vi "AssertXPathConnectorPanesMatchTemplateFiles.vi"(8 "error in (no error)":errorcluster, 9 "absolute custom device xml file":path, 10 "connector pane templates":T1[](array[typedef]), 11 "TestCase in":refnum<class "TestCase.lvclass">) -> (0 "error out":errorcluster, 3 "TestCase out":refnum<class "TestCase.lvclass">)   [LabVIEW 2015, in "VeriStandTestCase.lvclass"]
uses:
  VeriStandTestCase.lvclass
  <vilib>/addons/_JKI Toolkits/VI Tester/TestCase.llb/TestCase.lvclass
  ConnectorPaneTemplate.ctl
  <vilib>/xml/Load XML File.vi
  <userlib>/_OpenG.lib/array/array.llb/Remove Duplicates from 1D Array (String)__ogtk.vi
  <vilib>/xml/Close Reference(Node).vi
  <vilib>/xml/NI_XML.lvlib
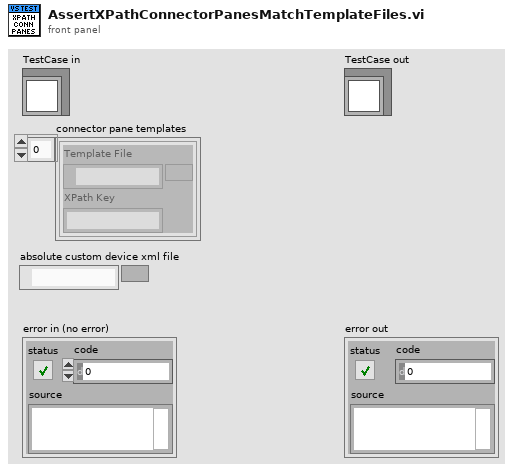
[diagram p1: front panel]
types:
  T1 = typedef "VeriStandTestCase.lvclass/ConnectorPaneTemplate.ctl" = cluster{"Template File":path, "XPath Key":string}
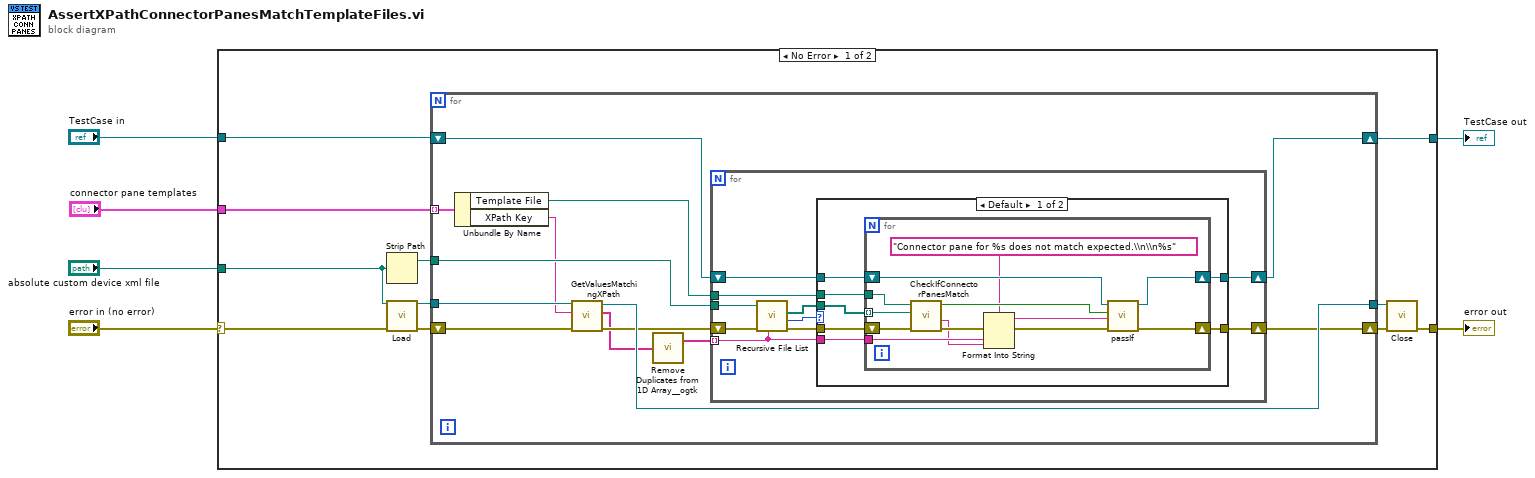
[diagram p0: block diagram]
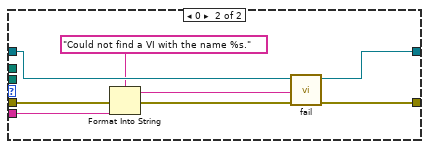
[diagram p2: hidden frame]
diagram:
  n1 = case shown="No Error" "error in (no error)" {
    selector: "error in (no error)" -> [w8 w70]
    tunnel: "absolute custom device xml file" -> [w16 _]
    tunnel: [w15 w69] -> w5
    tunnel: "TestCase in" -> [w13 w69]
    tunnel: [w11 w70] -> w3
    tunnel: "connector pane templates" -> [w7 _]
    frame No Error {
      n2 = Strip Path(path=w16) -> (stripped path=w17:path)  [unwired: 1 out]
      n3 = call-poly <vilib>:"Load.vi"("path to XML document"=w16, "error in (no error)"=w8) -> ("DOM document out"=w10:refnum<k20>, "error out"=w9:errorcluster)  [unwired: 11 in, 1 out]
      n4 = for {
        shift-right: [w23] -> w14
        shift-left: w9 -> [w29]
        tunnel: w10 -> [w30]
        tunnel: [w28] -> w12
        tunnel: w7 -> [w20] mode=indexing
        shift-right: [w27] -> w15
        shift-left: w13 -> [w26]
        tunnel: w17 -> [w25]
        n5 = Unbundle By Name(w20) -> ("Template File"=w18:path, "XPath Key"=w19:string)
        n6 = call "GetValuesMatchingXPath.vi"("error in (no error)"=w29, "XPath"=w19, "XML refnum in"=w30) -> ("error out"=w24:errorcluster, "Values"=w22:string[], "XML refnum out"=w28:refnum<k20>)  [unwired: 6 in]
        n7 = call-poly <userlib>:"Remove Duplicates from 1D Array__ogtk.vi"("Input Array"=w22) -> ("Output Array"=w21:string[])  [unwired: 1 out]
        n8 = for {
          shift-right: [w38] -> w23
          shift-left: w24 -> [w40]
          tunnel: w21 -> [w34] mode=indexing
          tunnel: w25 -> [w39]
          tunnel: w18 -> [w37]
          shift-right: [w35] -> w27
          shift-left: w26 -> [w36]
          n9 = call <vilib>:"Recursive File List.vi"("pattern"=w34, "error in (no error)"=w40, "Folder Path"=w39) -> ("error out"=w32:errorcluster, "Number of Files"=w33:i32, "All Files in Dir"=w31:path[])  [unwired: 4 in, 2 out]
          n10 = case shown="Default" w33 {
            tunnel: w32 -> [w47 w64]
            tunnel: [w45 w68] -> w38
            tunnel: w31 -> [w42 _]
            tunnel: w37 -> [w46 _]
            tunnel: w36 -> [w44 w67]
            tunnel: [w43 w66] -> w35
            tunnel: w34 -> [w41 w65]
            frame Default {
              n11 = for {
                tunnel: w46 -> [w59]
                shift-right: [w57] -> w45
                shift-left: w47 -> [w60]
                shift-right: [w55] -> w43
                shift-left: w44 -> [w56]
                tunnel: w42 -> [w54] mode=indexing
                tunnel: w41 -> [w52]
                n12 = call "CheckIfConnectorPanesMatch.vi"("error in (no error)"=w60, "actual connector pane vi"=w54, "expected connector pane vi"=w59) -> ("error out"=w50:errorcluster, "mismatch explanation"=w48:string, "connector panes match"=w58:bool)  [unwired: 6 in]
                n13 = Format Into String(format string="Connector pane for %s does not match expected.\\n\\n%s" ("connector pane mismatch error"), error in=w50, w52, w48) -> (resulting string=w51:string, error out=w53:errorcluster)  [unwired: 1 in]
                n14 = call-dynamic "passIf.vi"("error in (no error)"=w53, "message (\"\")"=w51, "pass"=w58, "TestCase in"=w56) -> ("error out"=w57:errorcluster, "TestCase out"=w55:refnum<class "TestCase.lvclass">)  [unwired: 6 in]
              }
            }
            frame 0 {
              n15 = Format Into String(format string="Could not find a VI with the name %s." ("no matches error"), error in=w64, w65) -> (resulting string=w62:string, error out=w63:errorcluster)  [unwired: 1 in]
              n16 = call-dynamic "fail.vi"("error in (no error)"=w63, "message (\"\")"=w62, "TestCase in"=w67) -> ("error out"=w68:errorcluster, "TestCase out"=w66:refnum<class "TestCase.lvclass">)  [unwired: 7 in]
            }
          }
        }
      }
      n17 = call-poly <vilib>:"Close.vi"("error in (no error)"=w14, "node"=w12) -> ("error out"=w11:errorcluster)  [unwired: 7 in]
    }
    frame Error {
    }
  }
  "TestCase out" <- w5
  "error out" <- w3
